vi "Set ID.vi"(10 "ID":i32, 11 "Thread in":refnum<class "Thread.lvclass">) -> (3 "Thread out":refnum<class "Thread.lvclass">)   [LabVIEW 2019, in "DSF Core.lvlib" / "Thread.lvclass"]
uses:
  Thread.lvclass
  Thread.lvclass/Thread.ctl
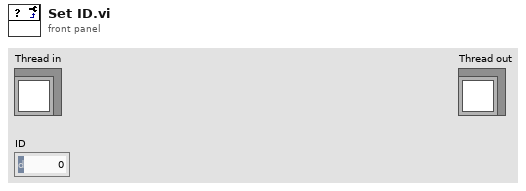
[diagram p1: front panel]
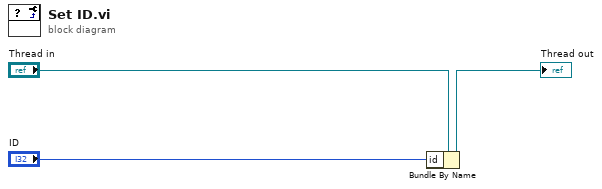
[diagram p0: block diagram]
diagram:
  n1 = Bundle By Name(cluster="Thread in", "id"="ID") -> (→"Thread out":refnum<class "Thread.lvclass">)
